vi "NI_Doppler_Digital.vi"() -> ()   [LabVIEW 2020]
panel:
  out "error out":errorcluster
  out "Waveform Graph":dynamicdata(graph)
  in  "stop (F)":bool
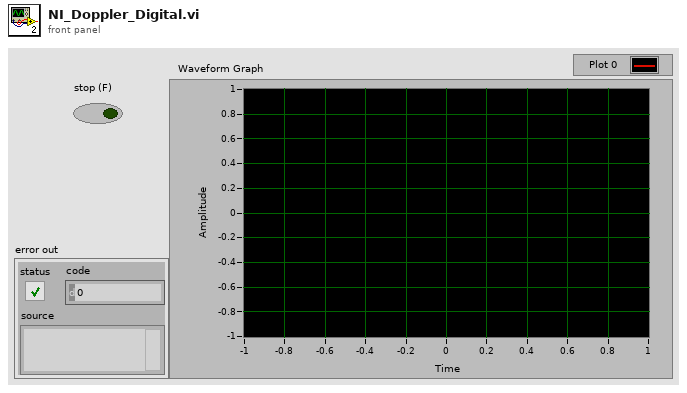
[diagram p1: front panel]
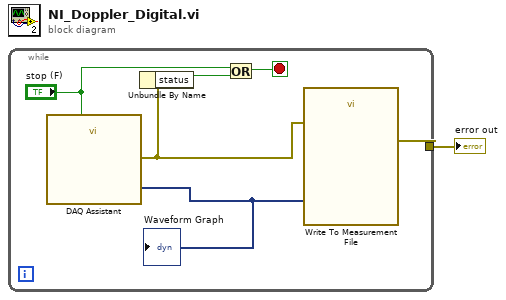
[diagram p0: block diagram]
diagram:
  n1 = while {
    tunnel: [w6] -> w1
    stop <- w5 stop-if-true
    n2 = call "DAQ Assistant"("stop (F)"="stop (F)") -> ("data"=w7:dynamicdata, "error out"=w2:errorcluster)  [unwired: 15 in, 2 out]
    "Waveform Graph" <- w7
    n3 = Unbundle By Name(w2) -> ("status"=w3:bool)
    n4 = Or(x="stop (F)", y=w3) -> (x .or. y?=w5:bool)
    n5 = call "Write To Measurement File"("Signals"=w7, "error in (no error)"=w2) -> ("error out"=w6:errorcluster)  [unwired: 15 in, 2 out]
  }
  "error out" <- w1
